vi "Check if Custom Device Enabled.vi"(8 "error in":errorcluster, 11 "custom device ref":T1 format="%.0x") -> (0 "error out":errorcluster, 2 "is enabled?":bool, 3 "custom device ref out":T1 format="%.0x")   [LabVIEW 2020, in "AIM MIL-STD-1553 Scripting.lvlib"]
uses:
  AIM MIL-STD-1553 Scripting.lvlib
  <vilib>/NI VeriStand/Custom Device API/Custom Device Item Ref.ctl
  Constants.vi
  <vilib>/NI VeriStand/Custom Device API/Custom Device API.lvlib
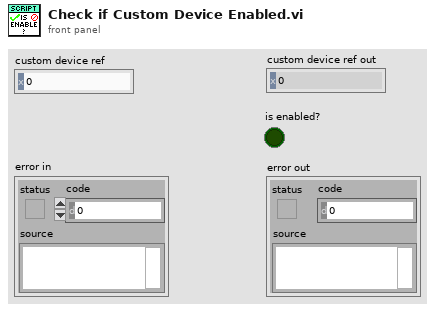
[diagram p1: front panel]
types:
  T1 = typedef "Custom Device API.lvlib/Custom Device Item Ref.ctl" = u64
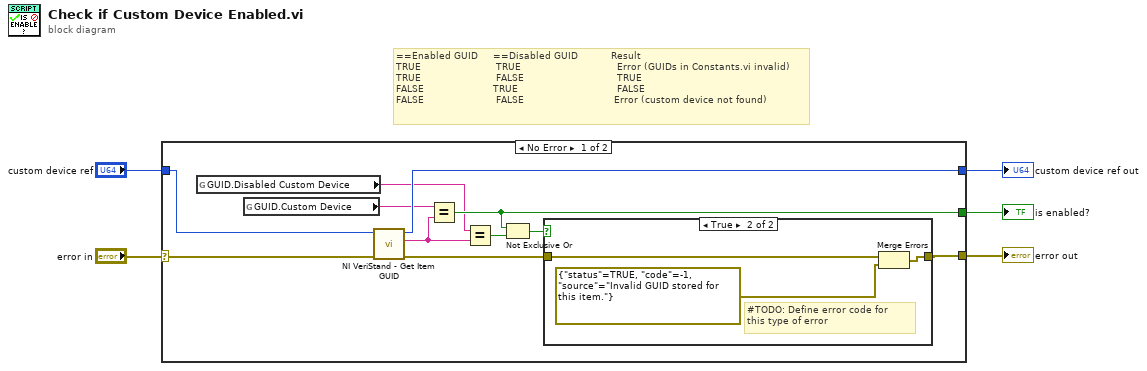
[diagram p0: block diagram]
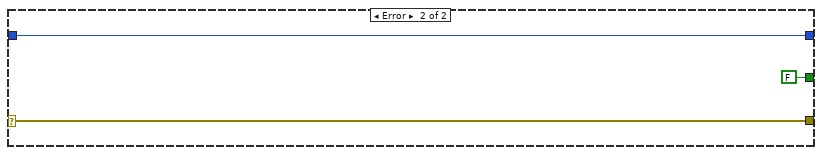
[diagram p3: hidden frame]
diagram:
  # "==Enabled GUID     ==Disabled GUID           Result\nTRUE                         TRUE                                Error (GUIDs in Constants.vi invalid)\nTRUE                         FALSE                               TRUE\nFALSE                       TRUE                                 FALSE\nFALSE                        FALSE                              Error (custom device not found)"
  n1 = case shown="No Error" "error in" {
    selector: "error in" -> [w16 w23]
    tunnel: [w14 w23] -> w4
    tunnel: [w12 w22] -> w3
    tunnel: "custom device ref" -> [w13 w22]
    tunnel: [w8 FALSE] -> w1
    frame No Error {
      n2 = global read "Constants.vi" "GUID.Disabled Custom Device"() -> (w6:string)
      n3 = global read "Constants.vi" "GUID.Custom Device"() -> (w7:string)
      n4 = call <vilib>:"NI VeriStand - Get Item GUID.vi"("error in (no error)"=w16, "Item Ref in"=w13) -> ("error out"=w15:errorcluster, "GUID"=w11:string, "Item Ref out"=w12:T1)  [unwired: 7 in]
      n5 = Equal?(x=w7, y=w11) -> (x = y?=w8:bool)
      n6 = Equal?(x=w6, y=w11) -> (x = y?=w9:bool)
      n7 = Not Exclusive Or(1:w9, 2:w8) -> (0:w10:bool)
      n8 = case shown="True" w10 {
        tunnel: [w17 w19] -> w14
        tunnel: w15 -> [w17 w18]
        frame False {
        }
        frame True {
          # "#TODO: Define error code for\nthis type of error"
          n9 = Merge Errors(w18, errorcluster {"status"=TRUE, "code"=-1, "source"="Invalid GUID stored for this item."} ("New Error")) -> (w19:errorcluster)
        }
      }
    }
    frame Error {
    }
  }
  "custom device ref out" <- w3
  "error out" <- w4
  "is enabled?" <- w1
